vi "water level indicator.vi"() -> ()   [LabVIEW 2025]
panel:
  out "water level":dbl
  out "water level is less":bool
  out "water level is more":bool
  in  "Knob":dbl(knob) scale=0.0..10.0
  out "Tank":dbl(slide) scale=0.0..10.0
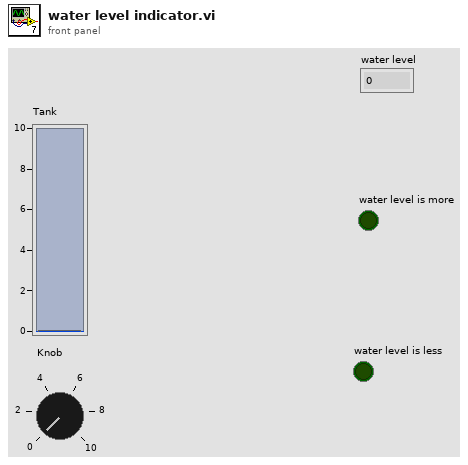
[diagram p1: front panel]
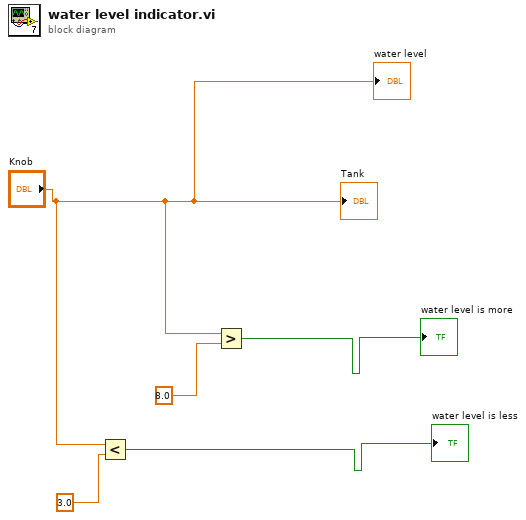
[diagram p0: block diagram]
diagram:
  n1 = Less?(x="Knob", y=3.0) -> (x < y?=→"water level is less":bool)
  n2 = Greater?(x="Knob", y=8.0) -> (0:→"water level is more":bool)
  "Tank" <- "Knob"
  "water level" <- "Knob"
